vi "Get Selection Event.vi"(11 "AutoComplete in":refnum<class "AutoComplete.lvclass">) -> (2 "Selection Event":refnum<user-event>)   [LabVIEW 2020, in "AutoComplete.lvlib" / "AutoComplete.lvclass"]
doc: "Gets the event that can be registered for to receive the selected string value when a user finishes an autocomplete selection."
uses:
  AutoComplete.lvclass
  AutoComplete.lvclass/AutoComplete.ctl
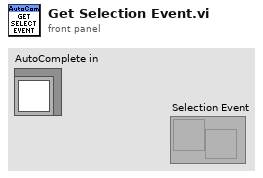
[diagram p1: front panel]
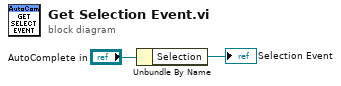
[diagram p0: block diagram]
diagram:
  n1 = Unbundle By Name("AutoComplete in") -> ("Selection"=→"Selection Event":refnum<user-event>)
